vi "RTS Extract Setup Single.vi"(8 "Error In":errorcluster, 9 "Station Number":u8=1 min=1 max=8 step=1, 10 "File Setup Data":string[][](array[string]), 11 "Station Settings In in":T1) -> (0 "Error Out":errorcluster, 2 "Updated Array":string[][](array[string]), 3 "Station Settings In out":T1)   [LabVIEW 2020]
uses:
  Type Definitions/RTS Station Settions TCP Comms.ctl
  Type Definitions/RTS Chamber Save Status.ctl
  Type Definitions/RTS Test Pattern.ctl
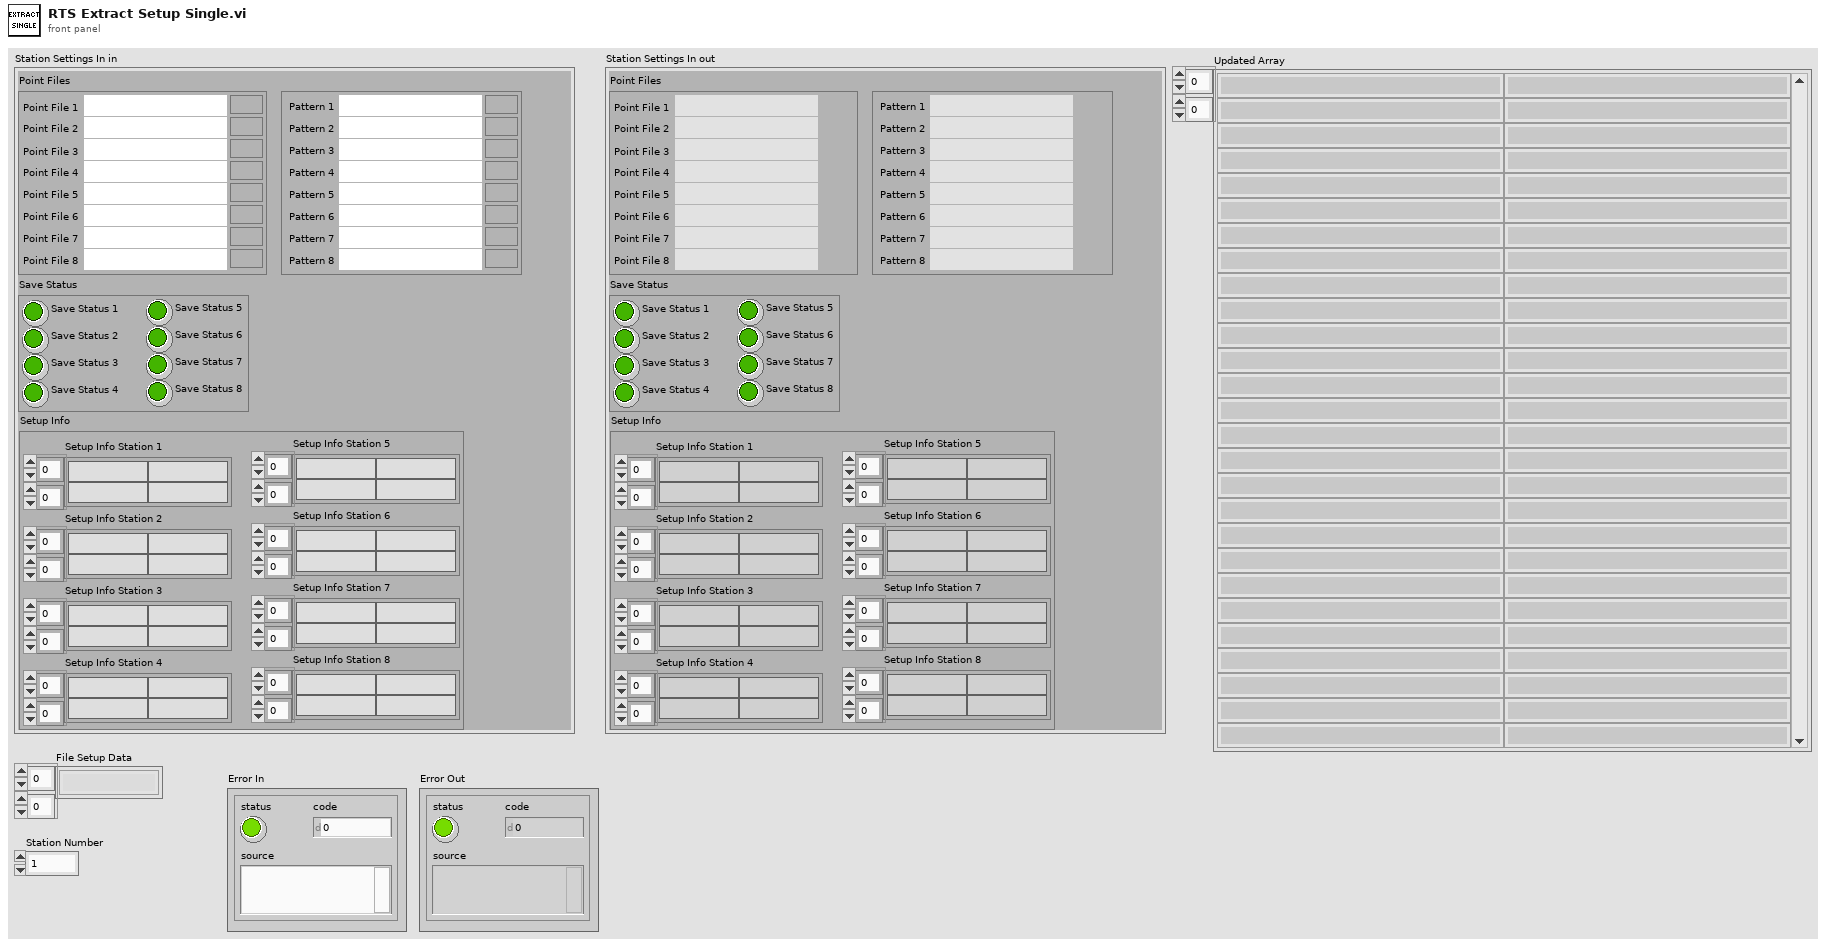
[diagram p1: front panel]
types:
  T1 = typedef "RTS Station Settions TCP Comms.ctl" = cluster{"Point Files":cluster{"Point File 1":path, "Point File 2":path, "Point File 3":path, "Point File 4":path, "Point File 5":path, "Point File 6":path, "Point File 7":path, "Point File 8":path}, "Save Status":T2, "Setup Info":cluster{"Setup Info Station 1":string[][], "Setup Info Station 2":string[][], "Setup Info Station 3":string[][], "Setup Info Station 4":string[][], "Setup Info Station 5":string[][], "Setup Info Station 6":string[][], "Setup Info Station 7":string[][], "Setup Info Station 8":string[][]}, "Chamber Test Pattern":T3}
  T2 = typedef "RTS Chamber Save Status.ctl" = cluster{"Save Status 1":bool, "Save Status 2":bool, "Save Status 3":bool, "Save Status 4":bool, "Save Status 5":bool, "Save Status 6":bool, "Save Status 7":bool, "Save Status 8":bool}
  T3 = typedef "RTS Test Pattern.ctl" = cluster{" Pattern 1":path, "Pattern 2":path, "Pattern 3":path, "Pattern 4":path, "Pattern 5":path, "Pattern 6":path, "Pattern 7":path, "Pattern 8":path}
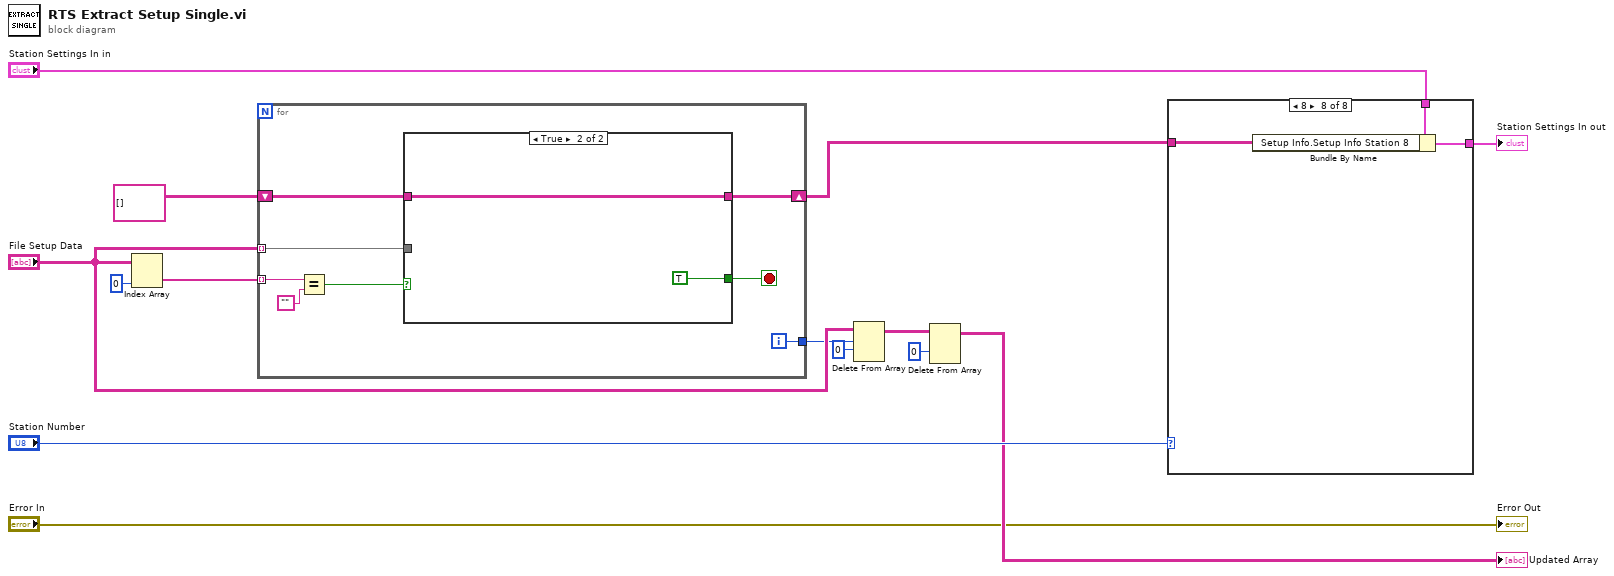
[diagram p0: block diagram]
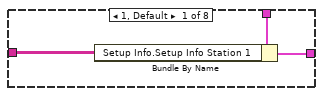
[diagram p2: hidden frame]
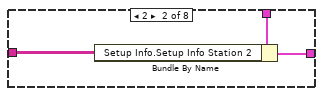
[diagram p3: hidden frame]
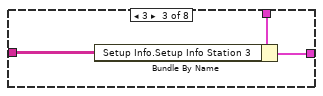
[diagram p4: hidden frame]
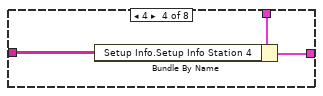
[diagram p5: hidden frame]
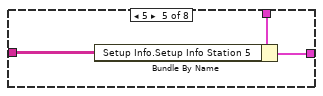
[diagram p6: hidden frame]
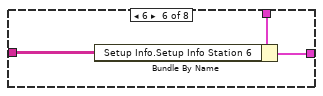
[diagram p7: hidden frame]
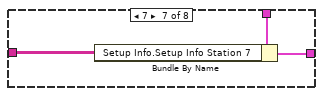
[diagram p8: hidden frame]
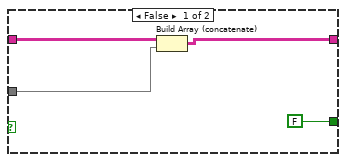
[diagram p9: hidden frame]
diagram:
  n1 = Index Array(array="File Setup Data", index (col)=0 ("disabled index (col)")) -> (element=w10:string[])  [unwired: 1 in]
  n2 = for {
    tunnel: w10 -> [w21] mode=indexing
    shift-right: [w19] -> w13
    shift-left: string[][] [] -> [w20]
    tunnel: "File Setup Data" -> [w16] mode=indexing
    tunnel: [w15] -> w6
    i -> [w15]
    stop <- w17 stop-if-true
    n3 = Equal?(x=w21, y="") -> (x = y?=w18:bool)
    n4 = case shown="True" w18 {
      tunnel: w20 -> [w25 w28]
      tunnel: [w24 w28] -> w19
      tunnel: [FALSE TRUE] -> w17
      tunnel: w16 -> [w23 _]
      frame False {
        n5 = Build Array (concatenate)(w25, w23) -> (w24:string[][])
      }
      frame True {
      }
    }
  }
  n6 = Delete From Array(array="File Setup Data", length=w6, index (row)=0) -> (array with subset deleted=w4:string[][])  [unwired: 1 in, 1 out]
  n7 = Delete From Array(array=w4, index (row)=0) -> (array with subset deleted=→"Updated Array":string[][])  [unwired: 2 in, 1 out]
  n8 = case shown="8" "Station Number" {
    tunnel: "Station Settings In in" -> [w31 w34 w37 w40 w43 w46 w49 w52]
    tunnel: w13 -> [w30 w32 w35 w38 w41 w44 w47 w50]
    tunnel: [w29 w33 w36 w39 w42 w45 w48 w51] -> w14
    frame 1, Default {
      n9 = Bundle By Name(cluster=w31, "Setup Info.Setup Info Station 1"=w30) -> (w29:T1)
    }
    frame 2 {
      n10 = Bundle By Name(cluster=w34, "Setup Info.Setup Info Station 2"=w32) -> (w33:T1)
    }
    frame 3 {
      n11 = Bundle By Name(cluster=w37, "Setup Info.Setup Info Station 3"=w35) -> (w36:T1)
    }
    frame 4 {
      n12 = Bundle By Name(cluster=w40, "Setup Info.Setup Info Station 4"=w38) -> (w39:T1)
    }
    frame 5 {
      n13 = Bundle By Name(cluster=w43, "Setup Info.Setup Info Station 5"=w41) -> (w42:T1)
    }
    frame 6 {
      n14 = Bundle By Name(cluster=w46, "Setup Info.Setup Info Station 6"=w44) -> (w45:T1)
    }
    frame 7 {
      n15 = Bundle By Name(cluster=w49, "Setup Info.Setup Info Station 7"=w47) -> (w48:T1)
    }
    frame 8 {
      n16 = Bundle By Name(cluster=w52, "Setup Info.Setup Info Station 8"=w50) -> (w51:T1)
    }
  }
  "Station Settings In out" <- w14
  "Error Out" <- "Error In"
